vi "set_node_attribute.vi"(7 "name":string, 8 "error in (no error)":errorcluster, 9 "value":variant, 10 "node":refnum<class "Node.lvclass">, 11 "graph":refnum<class "Graph.lvclass">) -> (0 "error out":errorcluster, 2 "replaced":bool, 3 "graph-out":refnum<class "Graph.lvclass">)   [LabVIEW 2020, in "graph.lvlib" / "Graph.lvclass"]
uses:
  Graph.lvclass
  Node/Node.lvclass
  Node/Node.lvclass/Node.ctl
  Graph.lvclass/Graph.ctl
  <vilib>/Utility/miscctls.llb/LVMapReplaceAction.ctl
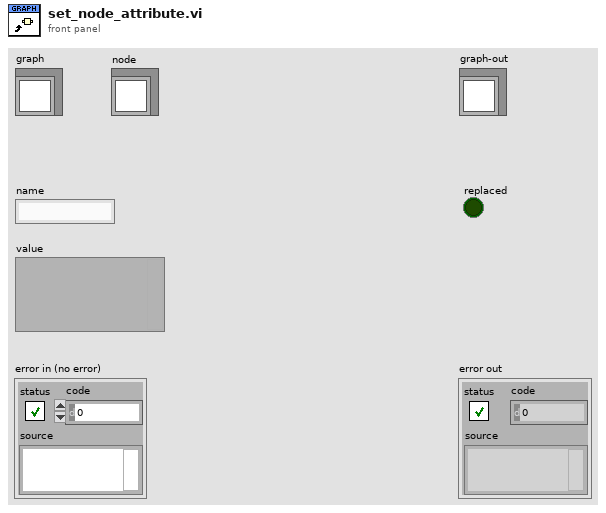
[diagram p1: front panel]
types:
  T1 = typedef "LVMapReplaceAction.ctl" = enum32{"Modify Entry only if found", "Add or Modify Entry", "Delete Entry"}
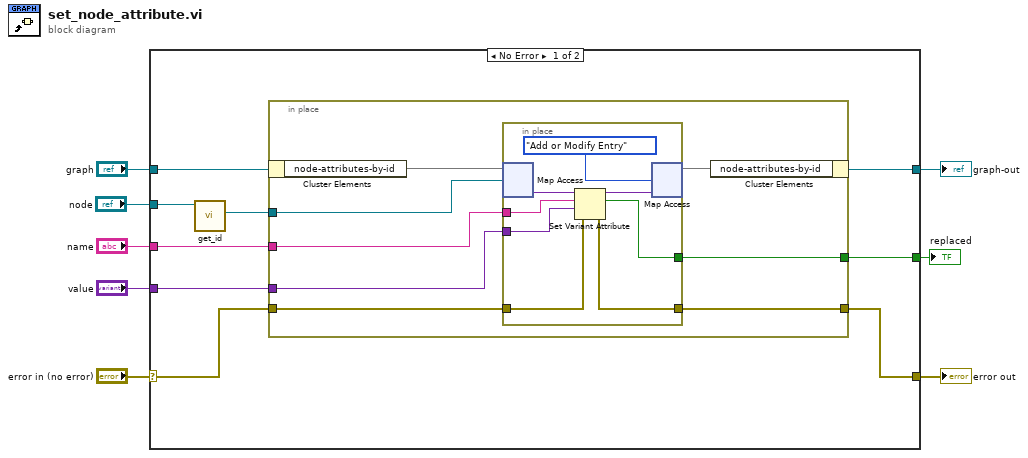
[diagram p0: block diagram]
diagram:
  n1 = case shown="No Error" "error in (no error)" {
    selector: "error in (no error)" -> [w13 w35]
    tunnel: [w12 w35] -> w7
    tunnel: [w15 w34] -> w5
    tunnel: "graph" -> [w14 w34]
    tunnel: "name" -> [w17 _]
    tunnel: "value" -> [w16 _]
    tunnel: "node" -> [w11 _]
    tunnel: [w9 _] -> w1
    frame No Error {
      n2 = call "get_id.vi"("node"=w11) -> ("node-id"=w10:refnum<class "ID.lvclass">)  [unwired: 10 in]
      n3 = in-place {
        in-place-border: w17 -> [w23]
        in-place-border: w16 -> [w22]
        in-place-border: w10 -> [w21]
        in-place-border: w13 -> [w20]
        in-place-border: [w19] -> w12
        in-place-border: [w18] -> w9
        n4 = in-place-cluster #1(w14) -> ("node-attributes-by-id"=w25:map{refnum<class "ID.lvclass">, variant})
        n5 = in-place {
          in-place-border: w23 -> [w31]
          in-place-border: w22 -> [w30]
          in-place-border: w20 -> [w28]
          in-place-border: [w27] -> w19
          in-place-border: [w26] -> w18
          n6 = in-place-map #2(w25, w21) -> (w33:variant)  [unwired: 1 in, 1 out]
          n7 = Set Variant Attribute(Variant=w33, name=w31, value=w30, error in=w28) -> (Variant out=w32:variant, replaced=w26:bool, error out=w27:errorcluster)
          n8 = in-place-map #2(w32, LVMapReplaceAction."Add or Modify Entry" ("action")) -> (w24:map{refnum<class "ID.lvclass">, variant})  [unwired: 2 out]
        }
        n9 = in-place-cluster #1("node-attributes-by-id"=w24) -> (w15:refnum<class "Graph.lvclass">)
      }
    }
    frame Error {
    }
  }
  "error out" <- w7
  "graph-out" <- w5
  "replaced" <- w1
